vi "Round 3 lock.vi"(8 "error in (no error)":errorcluster, 11 "KNR in":T1) -> (0 "error out":errorcluster, 3 "KNR out":T1)   [LabVIEW 2013]
uses:
  <userlib>/KNR OS 3.0 LabVIEW Toolkit/Type Definition/KNR3 Reference.ctl
  <userlib>/_FPGA Interface Advanced Tools/FPGA Interface Base/FPGA Interface Base.lvclass
  <userlib>/KNR OS 3.0 LabVIEW Toolkit/Type Definition/Resource.ctl
  <userlib>/KNR OS 3.0 LabVIEW Toolkit/Type Definition/DC Motor Port.ctl
  Global 1.vi
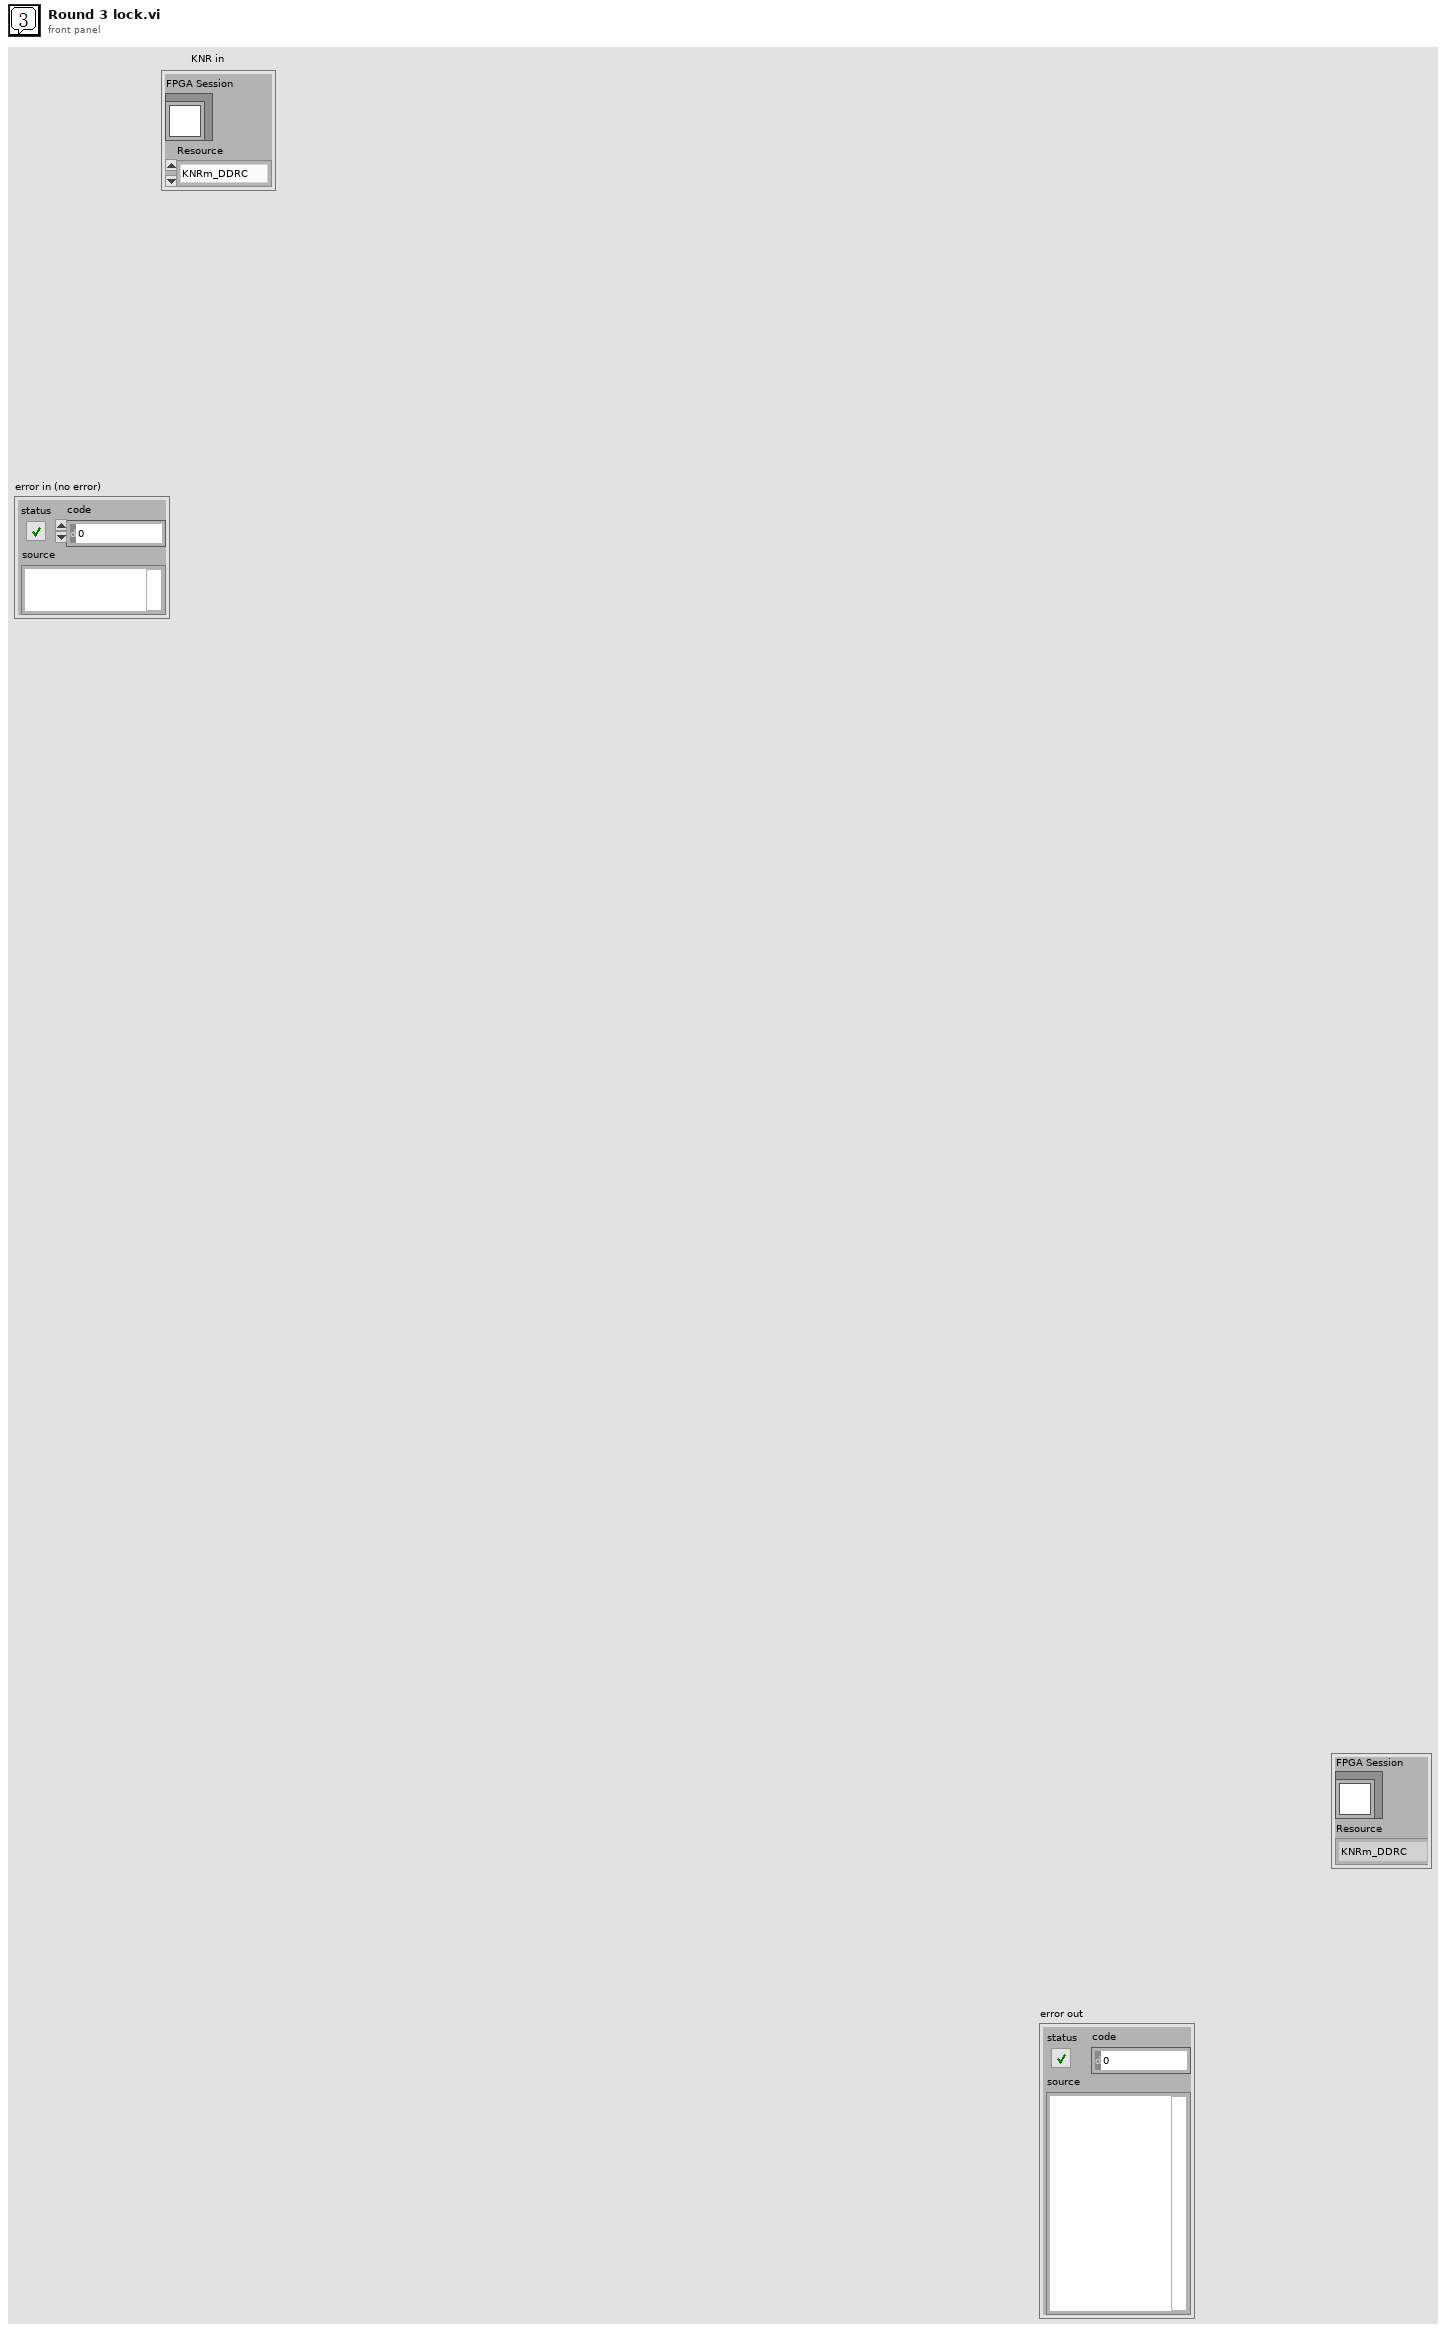
[diagram p1: front panel]
types:
  T1 = typedef "KNR3 Reference.ctl" = cluster{"FPGA Session":refnum<class "FPGA Interface Base.lvclass">, "Resource":T2}
  T2 = typedef "Resource.ctl" = enum16{"KNRm_DDRC", "KNRm_DDDD", "KNRm_DDDR", "KNRm_DDDC", "KNR"}
  T3 = typedef "DC Motor Port.ctl" = u16
  T4 = enum16{"white", "green", "left", "right", "C1", "C2"}
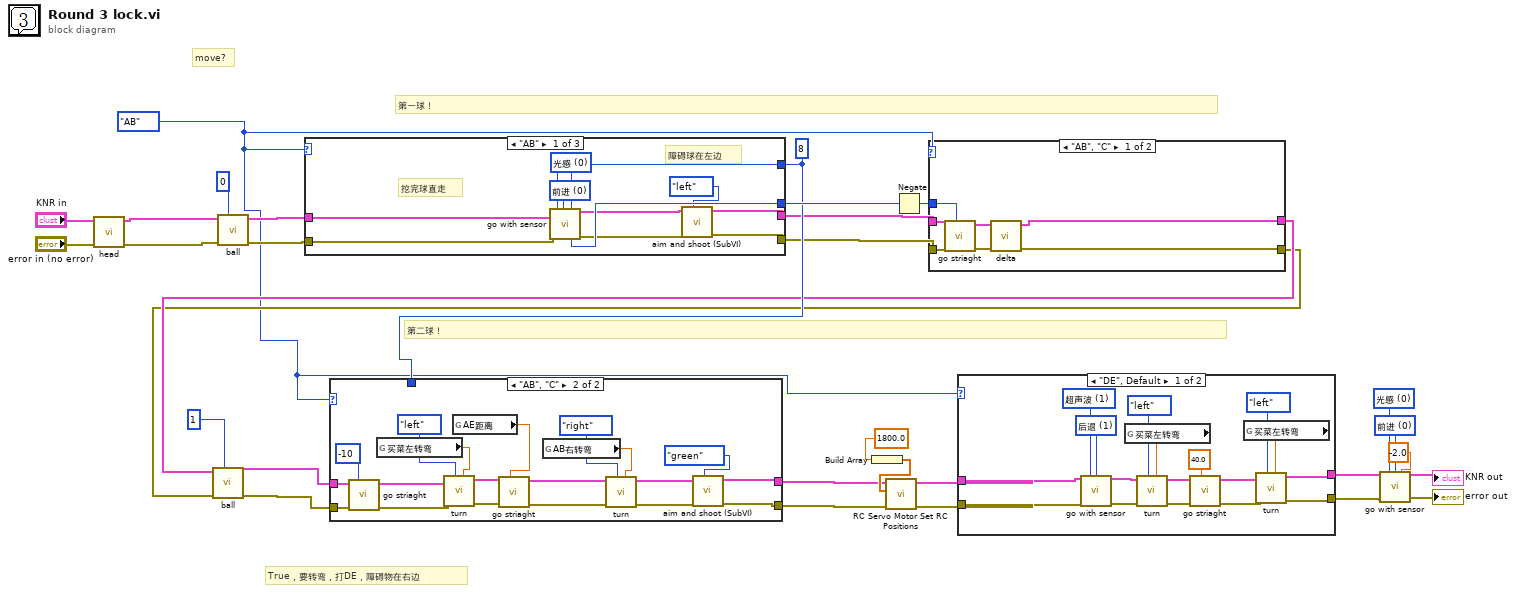
[diagram p0: block diagram]
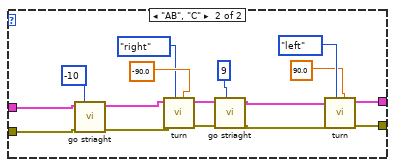
[diagram p2: hidden frame]
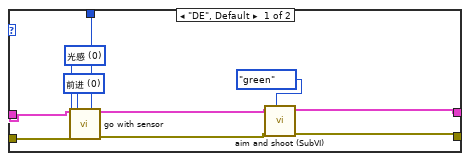
[diagram p3: hidden frame]
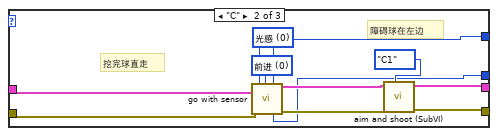
[diagram p4: hidden frame]
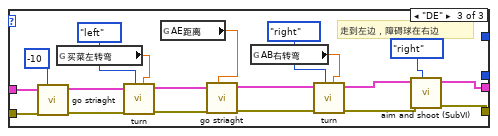
[diagram p5: hidden frame]
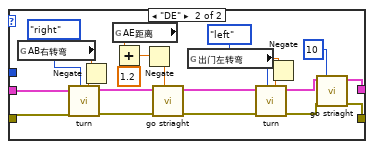
[diagram p6: hidden frame]
diagram:
  w1 = enum16{"DE", "AB", "C"}."AB" ("pin")
  w20 = 8
  w26 = T3 0 items=["前进", "后退"] ("方向")
  w27 = T3 0 items=["光感", "超声波"] ("传感器类型")
  # "True，要转弯，打DE，障碍物在右边"
  # "move?"
  # "第二球！"
  # "第一球！"
  n1 = call "head.vi"("error in (no error)"="error in (no error)", "KNR in"="KNR in") -> ("error out"=w2:errorcluster, "KNR out"=w3:T1)  [unwired: 8 in]
  n2 = call "ball.vi"("Numeric"=0, "error in (no error)"=w2, "KNR in"=w3) -> ("error out"=w19:errorcluster, "KNR out"=w24:T1)  [unwired: 6 in, 1 out]
  n3 = case shown="\"AB\"" w1 {
    tunnel: w24 -> [w40 w48 w61]
    tunnel: w19 -> [w39 w47 w60]
    tunnel: [w34 w46 w55] -> w10
    tunnel: [w32 w45 w54] -> w9
    tunnel: w20 -> [w38 w43 _]
    tunnel: [w37 w44 _] -> w21
    frame "AB" {
      w41 = T3 0 items=["前进", "后退"] ("方向")
      w42 = T3 0 items=["光感", "超声波"] ("传感器类型")
      # "障碍球在左边"
      # "挖完球直走"
      n4 = call "go with sensor.vi"("KNR in"=w40, "传感器类型"=w42, "方向"=w41, "then go:"=w38, "error in (no error)"=w39) -> ("KNR out"=w35:T1, "offset"=w37:i32, "error out"=w33:errorcluster)  [unwired: 8 in]
      n5 = call "aim and shoot (SubVI).vi"("pin"=enum16{"white", "green", "left", "right"}."left", "error in (no error)"=w33, "KNR in"=w35) -> ("error out"=w32:errorcluster, "KNR out"=w34:T1)  [unwired: 7 in]
    }
    frame "C" {
      w52 = T3 0 items=["前进", "后退"] ("方向")
      w53 = T3 0 items=["光感", "超声波"] ("传感器类型")
      # "障碍球在左边"
      # "挖完球直走"
      n6 = call "go with sensor.vi"("KNR in"=w48, "传感器类型"=w53, "方向"=w52, "then go:"=w43, "error in (no error)"=w47) -> ("KNR out"=w50:T1, "offset"=w44:i32, "error out"=w49:errorcluster)  [unwired: 8 in]
      n7 = call "aim and shoot (SubVI).vi"("pin"=T4."C1", "error in (no error)"=w49, "KNR in"=w50) -> ("error out"=w45:errorcluster, "KNR out"=w46:T1)  [unwired: 7 in]
    }
    frame "DE" {
      # "走到左边，障碍球在右边"
      n8 = call "go striaght.vi"("距离"=-10, "error in (no error)"=w60, "KNR in"=w61) -> ("error out"=w62:errorcluster, "KNR out"=w63:T1)  [unwired: 7 in]
      n9 = global read "Global 1.vi" "买菜左转弯"() -> (w71:dbl)
      n10 = call "turn.vi"("Angle"=w71, "side"=enum16{"right", "left"}."left", "error in (no error)"=w62, "KNR in"=w63) -> ("error out"=w64:errorcluster, "KNR out"=w65:T1)  [unwired: 6 in]
      n11 = global read "Global 1.vi" "AE距离"() -> (w68:dbl)
      n12 = call "go striaght.vi"("距离"=w68, "error in (no error)"=w64, "KNR in"=w65) -> ("error out"=w66:errorcluster, "KNR out"=w67:T1)  [unwired: 7 in]
      n13 = global read "Global 1.vi" "AB右转弯"() -> (w70:dbl)
      n14 = call "turn.vi"("Angle"=w70, "side"=enum16{"right", "left"}."right", "error in (no error)"=w66, "KNR in"=w67) -> ("error out"=w56:errorcluster, "KNR out"=w57:T1)  [unwired: 6 in]
      n15 = call "aim and shoot (SubVI).vi"("pin"=enum16{"white", "green", "left", "right"}."right", "error in (no error)"=w56, "KNR in"=w57) -> ("error out"=w54:errorcluster, "KNR out"=w55:T1)  [unwired: 7 in]
    }
  }
  n16 = Build Array(1800.0 ("element")) -> (w30:dbl[])
  n17 = Negate(x=w21) -> (-x=w22:i32)
  n18 = case shown="\"AB\", \"C\"" w1 {
    tunnel: [w74 w83] -> w17
    tunnel: [w73 w82] -> w16
    tunnel: w10 -> [w79 w92]
    tunnel: w9 -> [w78 w91]
    tunnel: w22 -> [w77 _]
    frame "AB", "C" {
      n19 = call "go striaght.vi"("距离"=w77, "error in (no error)"=w78, "KNR in"=w79) -> ("error out"=w76:errorcluster, "KNR out"=w75:T1)  [unwired: 7 in]
      n20 = call "delta.vi"("error in (no error)"=w76, "KNR in"=w75) -> ("error out"=w73:errorcluster, "KNR out"=w74:T1)  [unwired: 8 in]
    }
    frame "DE" {
      n21 = global read "Global 1.vi" "AB右转弯"() -> (w100:dbl)
      n22 = Negate(x=w100) -> (-x=w98:dbl)
      n23 = call "turn.vi"("Angle"=w98, "side"=enum16{"right", "left"}."right", "error in (no error)"=w91, "KNR in"=w92) -> ("error out"=w96:errorcluster, "KNR out"=w97:T1)  [unwired: 6 in]
      n24 = global read "Global 1.vi" "AE距离"() -> (w86:dbl)
      n25 = Add(x=w86, y=1.2) -> (x+y=w85:dbl)
      n26 = Negate(x=w85) -> (-x=w88:dbl)
      n27 = call "go striaght.vi"("距离"=w88, "error in (no error)"=w96, "KNR in"=w97) -> ("error out"=w93:errorcluster, "KNR out"=w94:T1)  [unwired: 7 in]
      n28 = global read "Global 1.vi" "出门左转弯"() -> (w90:dbl)
      n29 = Negate(x=w90) -> (-x=w89:dbl)
      n30 = call "turn.vi"("Angle"=w89, "side"=enum16{"right", "left"}."left", "error in (no error)"=w93, "KNR in"=w94) -> ("error out"=w80:errorcluster, "KNR out"=w81:T1)  [unwired: 6 in]
      n31 = call "go striaght.vi"("距离"=10, "error in (no error)"=w80, "KNR in"=w81) -> ("error out"=w82:errorcluster, "KNR out"=w83:T1)  [unwired: 7 in]
    }
  }
  n32 = call "ball.vi"("Numeric"=1, "error in (no error)"=w16, "KNR in"=w17) -> ("error out"=w4:errorcluster, "KNR out"=w18:T1)  [unwired: 6 in, 1 out]
  n33 = case shown="\"AB\", \"C\"" w1 {
    tunnel: w4 -> [w108 w117]
    tunnel: [w103 w114] -> w8
    tunnel: [w102 w112] -> w7
    tunnel: w20 -> [w107 _]
    tunnel: w18 -> [w101 w111]
    frame "DE", Default {
      w110 = T3 0 items=["前进", "后退"] ("方向")
      w109 = T3 0 items=["光感", "超声波"] ("传感器类型")
      n34 = call "go with sensor.vi"("KNR in"=w101, "传感器类型"=w109, "方向"=w110, "then go:"=w107, "error in (no error)"=w108) -> ("KNR out"=w105:T1, "error out"=w104:errorcluster)  [unwired: 8 in, 1 out]
      n35 = call "aim and shoot (SubVI).vi"("pin"=enum16{"white", "green", "left", "right"}."green", "error in (no error)"=w104, "KNR in"=w105) -> ("error out"=w102:errorcluster, "KNR out"=w103:T1)  [unwired: 7 in]
    }
    frame "AB", "C" {
      n36 = call "go striaght.vi"("距离"=-10, "error in (no error)"=w117, "KNR in"=w111) -> ("error out"=w118:errorcluster, "KNR out"=w119:T1)  [unwired: 7 in]
      n37 = global read "Global 1.vi" "买菜左转弯"() -> (w128:dbl)
      n38 = call "turn.vi"("Angle"=w128, "side"=enum16{"right", "left"}."left", "error in (no error)"=w118, "KNR in"=w119) -> ("error out"=w121:errorcluster, "KNR out"=w122:T1)  [unwired: 6 in]
      n39 = global read "Global 1.vi" "AE距离"() -> (w125:dbl)
      n40 = call "go striaght.vi"("距离"=w125, "error in (no error)"=w121, "KNR in"=w122) -> ("error out"=w123:errorcluster, "KNR out"=w124:T1)  [unwired: 7 in]
      n41 = global read "Global 1.vi" "AB右转弯"() -> (w127:dbl)
      n42 = call "turn.vi"("Angle"=w127, "side"=enum16{"right", "left"}."right", "error in (no error)"=w123, "KNR in"=w124) -> ("error out"=w113:errorcluster, "KNR out"=w115:T1)  [unwired: 6 in]
      n43 = call "aim and shoot (SubVI).vi"("pin"=enum16{"white", "green", "left", "right"}."green", "error in (no error)"=w113, "KNR in"=w115) -> ("error out"=w112:errorcluster, "KNR out"=w114:T1)  [unwired: 7 in]
    }
  }
  n44 = call <userlib>:"RC Servo Motor Set RC Positions.vi"("error in (no error)"=w7, "RC Pulse Width (1500 uS)"=w30, "KNR in"=w8) -> ("error out"=w28:errorcluster, "KNR out"=w29:T1)  [unwired: 7 in]
  n45 = case shown="\"DE\", Default" w1 {
    tunnel: w29 -> [w144 w150]
    tunnel: w28 -> [w143 w147]
    tunnel: [w131 w156] -> w6
    tunnel: [w130 w155] -> w5
    frame "DE", Default {
      w145 = T3 1 items=["前进", "后退"] ("方向")
      w146 = T3 1 items=["光感", "超声波"] ("传感器类型")
      n46 = call "go with sensor.vi"("KNR in"=w144, "传感器类型"=w146, "方向"=w145, "error in (no error)"=w143) -> ("KNR out"=w140:T1, "error out"=w139:errorcluster)  [unwired: 9 in, 1 out]
      n47 = global read "Global 1.vi" "买菜左转弯"() -> (w141:dbl)
      n48 = call "turn.vi"("Angle"=w141, "side"=enum16{"right", "left"}."left", "error in (no error)"=w139, "KNR in"=w140) -> ("error out"=w138:errorcluster, "KNR out"=w137:T1)  [unwired: 6 in]
      n49 = call "go striaght.vi"("距离"=40.0, "error in (no error)"=w138, "KNR in"=w137) -> ("error out"=w132:errorcluster, "KNR out"=w133:T1)  [unwired: 7 in]
      n50 = global read "Global 1.vi" "买菜左转弯"() -> (w134:dbl)
      n51 = call "turn.vi"("Angle"=w134, "side"=enum16{"right", "left"}."left", "error in (no error)"=w132, "KNR in"=w133) -> ("error out"=w130:errorcluster, "KNR out"=w131:T1)  [unwired: 6 in]
    }
    frame "AB", "C" {
      n52 = call "go striaght.vi"("距离"=-10, "error in (no error)"=w147, "KNR in"=w150) -> ("error out"=w148:errorcluster, "KNR out"=w149:T1)  [unwired: 7 in]
      n53 = call "turn.vi"("Angle"=-90.0, "side"=enum16{"right", "left"}."right", "error in (no error)"=w148, "KNR in"=w149) -> ("error out"=w158:errorcluster, "KNR out"=w159:T1)  [unwired: 6 in]
      n54 = call "go striaght.vi"("距离"=9, "error in (no error)"=w158, "KNR in"=w159) -> ("error out"=w153:errorcluster, "KNR out"=w154:T1)  [unwired: 7 in]
      n55 = call "turn.vi"("Angle"=90.0, "side"=enum16{"right", "left"}."left", "error in (no error)"=w153, "KNR in"=w154) -> ("error out"=w155:errorcluster, "KNR out"=w156:T1)  [unwired: 6 in]
    }
  }
  n56 = call "go with sensor.vi"("KNR in"=w6, "传感器类型"=w27, "方向"=w26, "then go:"=-2.0, "error in (no error)"=w5) -> ("KNR out"=→"KNR out":T1, "error out"=→"error out":errorcluster)  [unwired: 8 in, 1 out]
